vi "top_temperature.vi"() -> ()   [LabVIEW 2014]
panel:
  in  "stop":bool
  out "Waveform Chart":dbl(graph)
  in  "winter upper bound":dbl
  in  "winter lower bound":dbl
  in  "summer / winter":bool
  in  "Celsius / Fahrenheit":bool
  in  "summer upper bound":dbl
  in  "summer lower bound":dbl
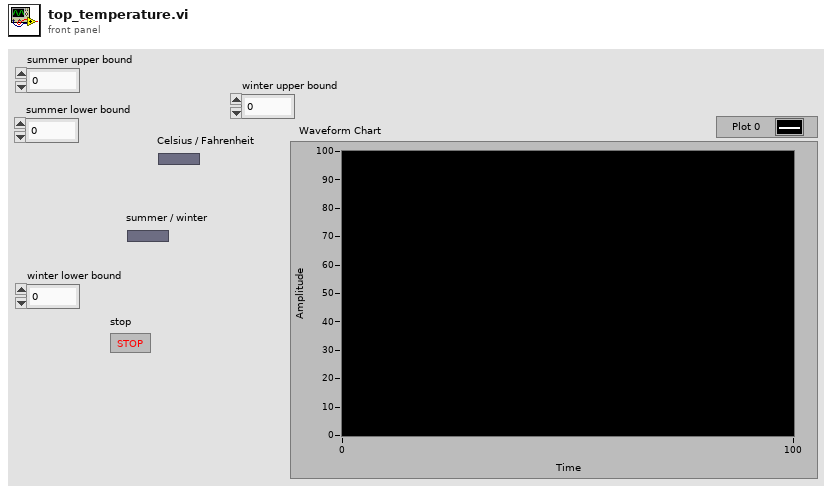
[diagram p1: front panel]
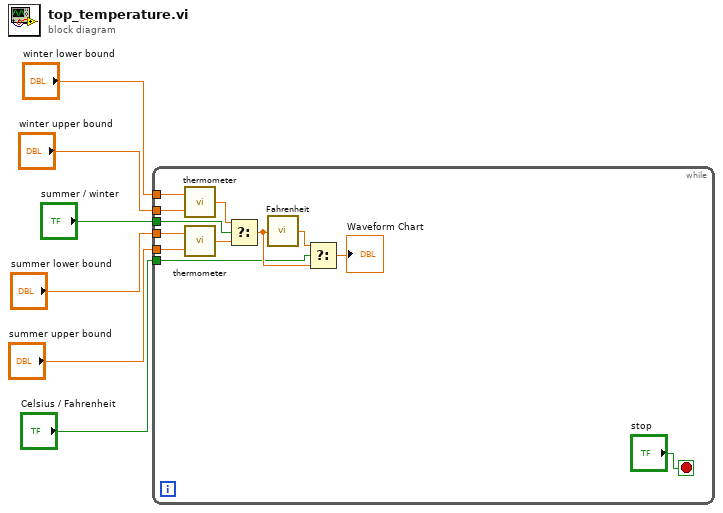
[diagram p0: block diagram]
diagram:
  n1 = while {
    tunnel: "winter lower bound" -> [w12]
    tunnel: "winter upper bound" -> [w11]
    tunnel: "summer lower bound" -> [w10]
    tunnel: "summer upper bound" -> [w9]
    tunnel: "Celsius / Fahrenheit" -> [w8]
    tunnel: "summer / winter" -> [w7]
    stop <- "stop" stop-if-true
    n2 = call "thermometer.vi"("upper bound"=w11, "lower bound"=w12) -> ("Deg C"=w15:dbl)
    n3 = call "thermometer.vi"("upper bound"=w9, "lower bound"=w10) -> ("Deg C"=w14:dbl)
    n4 = Select(t=w15, s=w7, f=w14) -> (s? t:f=w18:dbl)
    n5 = call "Fahrenheit.vi"("Deg C"=w18) -> ("Deg F"=w17:dbl)
    n6 = Select(t=w17, s=w8, f=w18) -> (s? t:f=→"Waveform Chart":dbl)
  }
